vi "NextState.vi"(0 "object in":refnum<class "InterceptPassTactic_v2.lvclass">, 2 "Robot in":refnum<class "Robot.lvclass">, 4 "GameRef":refnum<data-value>, 5 "error in (no error)":errorcluster) -> (14 "object out":refnum<class "InterceptPassTactic_v2.lvclass">, 19 "error out":errorcluster)   [LabVIEW 2023, in "InterceptPassTactic_v2.lvclass"]
uses:
  InterceptPassTactic_v2.lvclass
  C:/Users/ebert/Documents/codes/SSL/repo/SSL_AI/NewSTP/NewTactics/Tactic_v2_class/Tactic_v2.lvclass
  Robot_class/Robot.lvclass
  Game_class/Game.lvclass
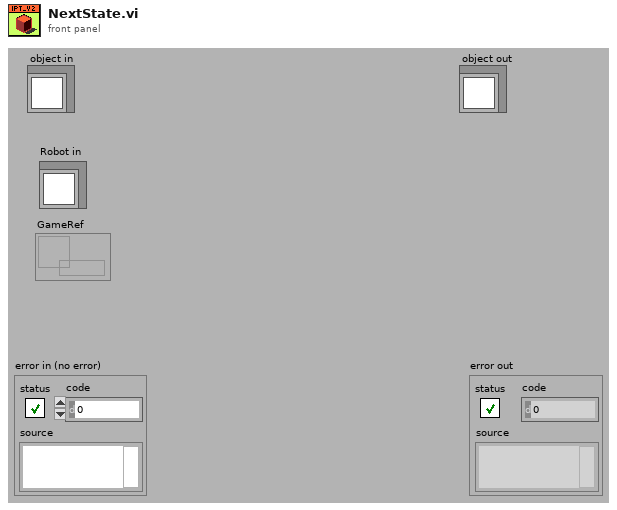
[diagram p1: front panel]
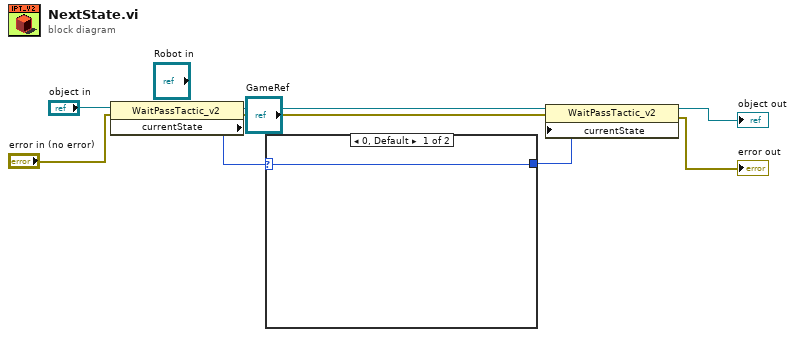
[diagram p0: block diagram]
diagram:
  n1 = property class="WaitPassTactic_v2"(reference="object in", error in="error in (no error)") -> (reference out=w6:refnum<class "InterceptPassTactic_v2.lvclass">, error out=w5:errorcluster, "currentState"=w8:u8)
  n2 = case shown="0, Default" w8 {
    selector: w8 -> [w9 w10]
    tunnel: [w9 w10] -> w7
    frame 0, Default {
    }
    frame 1 {
    }
  }
  n3 = property class="WaitPassTactic_v2"(reference=w6, error in=w5, "currentState"=w7) -> (reference out=→"object out":refnum<class "InterceptPassTactic_v2.lvclass">, error out=→"error out":errorcluster)
